vi "Deinitialize Dispenser.vi"(8 "error in (no error)":errorcluster, 11 "Gantry Class in":refnum<class "Gantry.lvclass">) -> (0 "error out":errorcluster, 3 "Gantry Class out":refnum<class "Gantry.lvclass">)   [LabVIEW 2017, in "Gantry.lvclass"]
uses:
  Gantry.lvclass
  Gantry.lvclass/Gantry.ctl
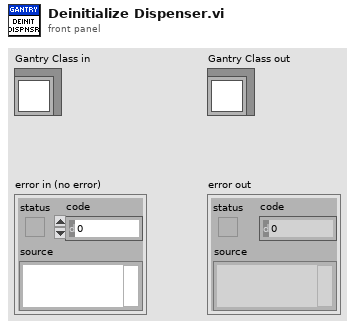
[diagram p1: front panel]
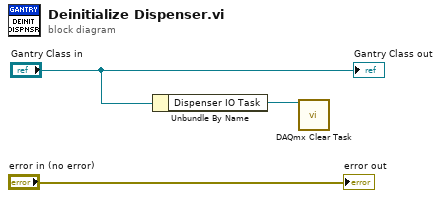
[diagram p0: block diagram]
diagram:
  n1 = Unbundle By Name("Gantry Class in") -> ("Dispenser IO Task"=w3:refnum<k21>)
  n2 = call <vilib>:"DAQmx Clear Task.vi"("task in"=w3) -> ()  [unwired: 14 in, 1 out]
  "error out" <- "error in (no error)"
  "Gantry Class out" <- "Gantry Class in"
